vi "APC_9056_ArControl.vi"(1 "LoadIni?":bool, 3 "input cluster":T3={"AR-FT-001"=nan, "O2-FC-001"=-1.1539459916321034e-07, "SW-FT-004"=7.081032221378816e-08, "SW-FT-002"=-4.7206881475858774e-08, "WF-OA-002"=0.4443584404854535, "WF-PT-004"=nan, "WF-OA-001"=0.4434660166344514, "EC-TT-001"=2293.7171636993767, "WF-TT-004"=2293.7171636993767, "EC-FC-001"=0.0, "NG-FC-001"=-6.294250863447837e-08, "EO-TT-001"=2293.5316367979103, "SW-FC-008"=nan, "SW-FC-004"=0.0, "IMEPn6"=1.91605028485912e-05, "TORQUE"=0.44243251168443165, "CylPresWarnings"=5.764607523039514e+17, "CylPresErrors"=0.0, "NG-FT-001"=-1.3899803990113974e-07, "EngineSpeed_rpm"=0.0}) -> (0 "AR-PC-002-REF":dbl format="%.2f")   [LabVIEW 2020]
uses:
  controls/APC_PIDCluster.ctl
  controls/APC_ControlSettings.ctl
  controls/APC_PIDcontrolSettings.ctl
  controls/APC_cascadePIDsettings.ctl
  <vilib>/addons/control/pid/pid.llb/PID Advanced (DBL).vi
  <vilib>/Utility/xml.llb/Read From XML File(string).vi
  <vilib>/Utility/xml.llb/Write to XML File(string).vi
  <vilib>/addons/control/pid/NI_PID_pid.lvlib
panel:
  in  "PC_ControlSettings":T1={"Spark advance [CADBTDC]"=0.0, "Pref"=0.0, "O2ref"=0.0, "DI advance [CADBTDC]"=0.0, "DI duration [ms] "=0.0, "CO2ref"=0.0, "PFI duration [ms]"=0.0, "IMEP ref"=0.0, "Speed ref"=1800.0, "IGN enable"=TRUE, "DI enable"=TRUE, "CL PFI\n lambda"=FALSE, "CL PFI\nIMEP"=FALSE, "Activate\ncylinder"=[FALSE, FALSE, FALSE, FALSE, FALSE, FALSE], "Force idling"=FALSE, "Force motoring"=FALSE, "ETP resync"=FALSE, "Requested mode"=0, "Clear Sync Errors"=FALSE, "toggle TDC"=FALSE, "l ref"=0.0, "PID control references"={"NG"=FALSE, "Ar"=FALSE, "O2"=FALSE, "Intake vent"=FALSE, "Cross vent"=FALSE, "Exhaust vent"=FALSE, "NG control mode"=0, "NG-FC-001-REF"=0.0, "WF-OA-002-REF"=0.0, "IMEP-REF"=0.0, "Nm-REF"=0.0, "Ar control mode"=0, "AR-PC-002-REF"=0.0, "WF-PT-004-REF"=0.0, "O2 control mode"=0, "O2-FC-001-REF"=0.0, "WF-OA-001-REF"=0.0, "Tcoolant control  mode"=0, "EC-FC-001-REF"=0.0, "EC-TT-001-REF"=0.0, "Texh control mode"=0, "SW-FC-004-REF"=0.0, "SW-FT-002-REF"=0.0, "WF-TT-004-REF"=0.0, "Toil control mode"=0, "SW-FC-009-REF"=0.0, "SW-FT-004-REF"=0.0, "EO-TT-001-REF"=0.0, "AIC201_CO2_ConcTarget"=0.0, "O2_FF_NG"=FALSE, "Dyno control mode"=0, "Membrane control mode"=0, "AR-FT-001-REF"=0.0, "MTR modbus floats"=[0.0, 0.0, 0.0, 0.0, 0.0, 0.0, 0.0, 0.0, 0.0, 0.0, 0.0, 0.0, 0.0, 0.0, 0.0, 0.0, 0.0, 0.0, 0.0], "MTR modbus u16"=[0, 0, 0, 0, 0, 0, 0], "MTR HB"=FALSE, "PC_HB"=FALSE, "EMERGENCY STOP"=FALSE}, "CA50setpoint [CADATDC]"=0.0, "CA50 control"=TRUE, "Knock control"=FALSE, "CLEAR EMERGENCY STOP"=FALSE, "EMERGENCY STOP"=FALSE}
  out "PID control references.Ar":bool
  out "direct?":bool
  in  "AR-PC-002-REF (manual)":dbl
  out "Direct control":dbl=50.0 format="%.2f"
  in  "save":bool
  in  "load":bool
  out "Ar control mode":u8=2
  out "AR-FT-001":dbl=-1.0490418105746395e-08
  in  "LL FF control":dbl format="%.2f"
  in  "reinitialize LL? (F)":bool
  out "WF-PT-004":dbl=2293.8148612417403
  in  "SW-FT-001-REF (manual)":dbl
  in  "WF-PT-004-REF (manual)":dbl
  in  "Ar control mode (manual)":u8
  out "HL on?":bool
  out "HL setpoint":dbl=400.0 format="%.2f"
  in  "LL PID gains":T4 {"derivative time (Td, min)" format="%.3f"; "integral time (Ti, min)" format="%.3f"; "proportional gain (Kc)" format="%.3f"}
  in  "LL PID setpoint range":cluster{"setpoint high":dbl, "setpoint low":dbl} {"setpoint high" format="%.2f"; "setpoint low" format="%.2f"}
  in  "LL PID output range":cluster{"output high":dbl, "output low":dbl} {"output low" format="%.2f"; "output high" format="%.2f"}
  in  "Override PC PID references":bool
  in  "HL learn?":bool
  in  "HL FF control":dbl format="%.2f"
  in  "HL PID gains":T4 {"derivative time (Td, min)" format="%.3f"; "integral time (Ti, min)" format="%.3f"; "proportional gain (Kc)" format="%.3f"}
  in  "HL PID setpoint range":cluster{"setpoint high":dbl, "setpoint low":dbl} {"setpoint high" format="%.2f"; "setpoint low" format="%.2f"}
  in  "HL PID output range":cluster{"output high":dbl, "output low":dbl} {"output low" format="%.2f"; "output high" format="%.2f"}
  in  "Safe mode control":dbl format="%.2f"
  in  "LL learn?":bool
  in  "reinitialize HL? (F)":bool
  out "LL on?":bool=TRUE
  out "LL setpoint":dbl=40.0 format="%.2f"
  # "Ar control"
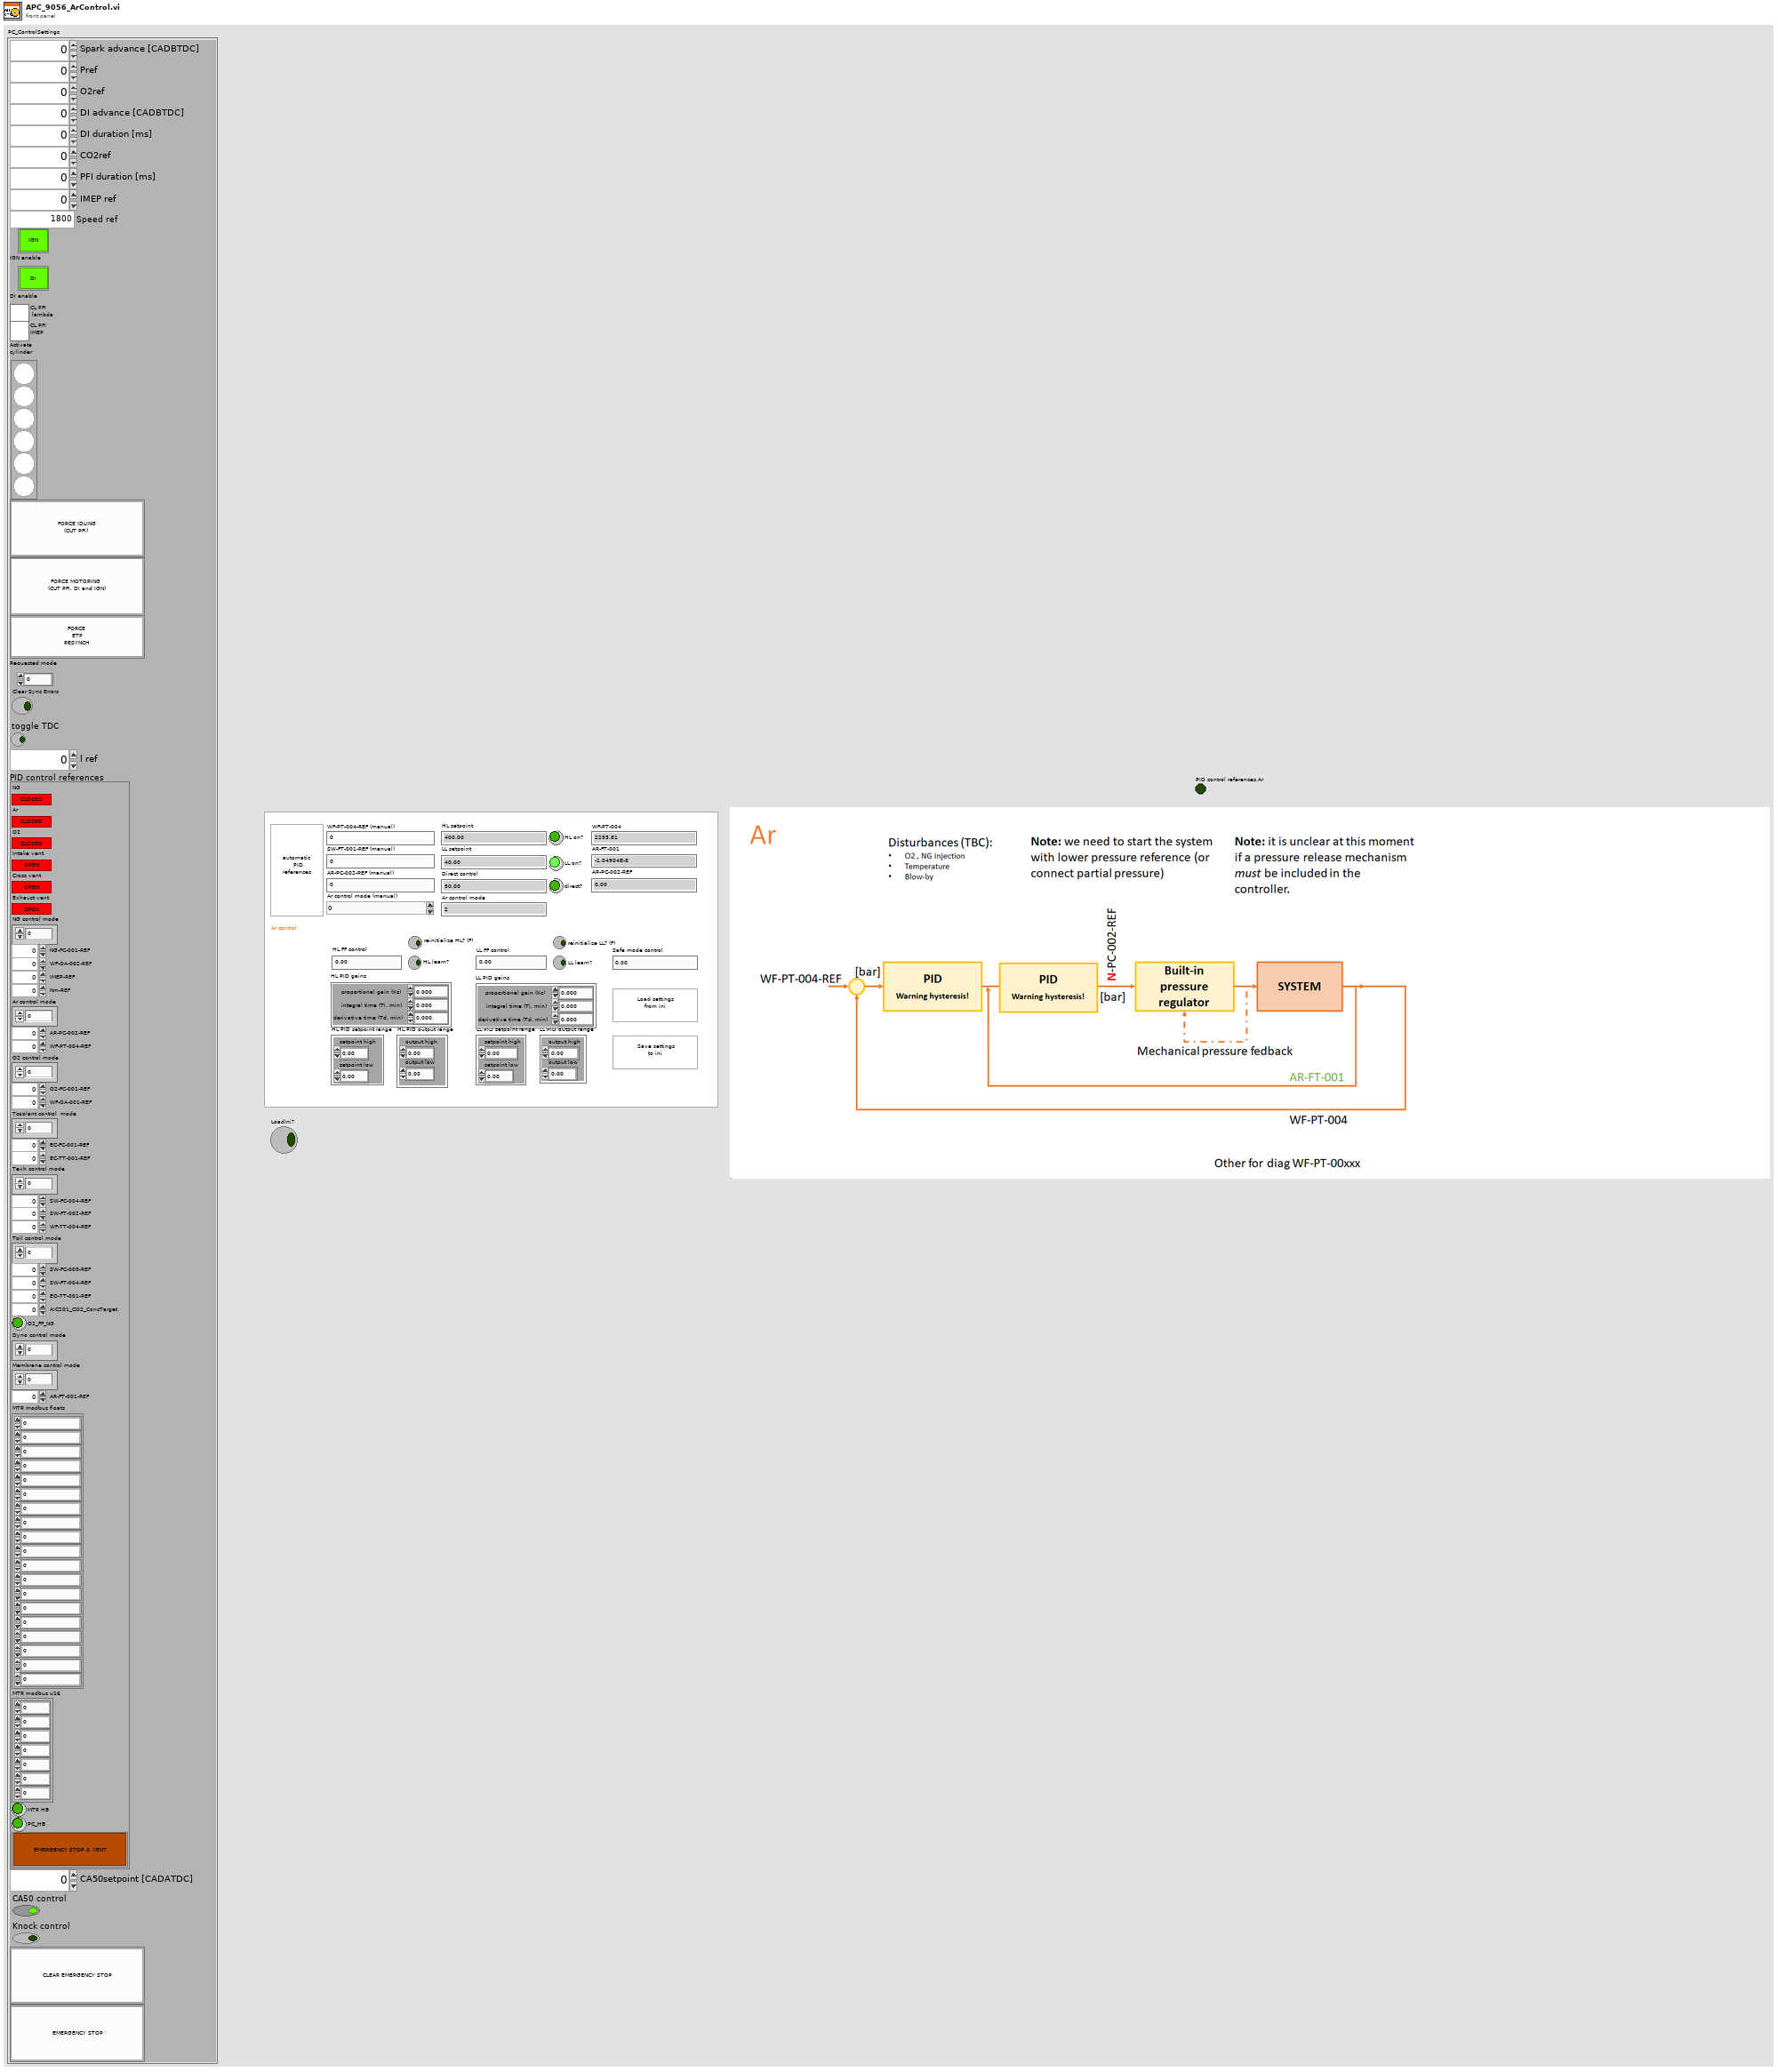
[diagram p1: front panel]
types:
  T1 = typedef "APC_ControlSettings.ctl" = cluster{"Spark advance [CADBTDC]":dbl, "Pref":dbl, "O2ref":dbl, "DI advance [CADBTDC]":dbl, "DI duration [ms] ":dbl, "CO2ref":dbl, "PFI duration [ms]":dbl, "IMEP ref":dbl, "Speed ref":dbl, "IGN enable":bool, "DI enable":bool, "CL PFI\n lambda":bool, "CL PFI\nIMEP":bool, "Activate\ncylinder":bool[], "Force idling":bool, "Force motoring":bool, "ETP resync":bool, "Requested mode":i8, "Clear Sync Errors":bool, "toggle TDC":bool, "l ref":dbl, "PID control references":T2, "CA50setpoint [CADATDC]":dbl, "CA50 control":bool, "Knock control":bool, "CLEAR EMERGENCY STOP":bool, "EMERGENCY STOP":bool}
  T2 = typedef "APC_PIDcontrolSettings.ctl" = cluster{"NG":bool, "Ar":bool, "O2":bool, "Intake vent":bool, "Cross vent":bool, "Exhaust vent":bool, "NG control mode":u8, "NG-FC-001-REF":dbl, "WF-OA-002-REF":dbl, "IMEP-REF":dbl, "Nm-REF":dbl, "Ar control mode":u8, "AR-PC-002-REF":dbl, "WF-PT-004-REF":dbl, "O2 control mode":u8, "O2-FC-001-REF":dbl, "WF-OA-001-REF":dbl, "Tcoolant control  mode":u8, "EC-FC-001-REF":dbl, "EC-TT-001-REF":dbl, "Texh control mode":u8, "SW-FC-004-REF":dbl, "SW-FT-002-REF":dbl, "WF-TT-004-REF":dbl, "Toil control mode":u8, "SW-FC-009-REF":dbl, "SW-FT-004-REF":dbl, "EO-TT-001-REF":dbl, "AIC201_CO2_ConcTarget":dbl, "O2_FF_NG":bool, "Dyno control mode":u8, "Membrane control mode":u8, "AR-FT-001-REF":dbl, "MTR modbus floats":sgl[], "MTR modbus u16":u16[], "MTR HB":bool, "PC_HB":bool, "EMERGENCY STOP":bool}
  T3 = typedef "APC_PIDCluster.ctl" = cluster{"AR-FT-001":dbl, "O2-FC-001":dbl, "SW-FT-004":dbl, "SW-FT-002":dbl, "WF-OA-002":dbl, "WF-PT-004":dbl, "WF-OA-001":dbl, "EC-TT-001":dbl, "WF-TT-004":dbl, "EC-FC-001":dbl, "NG-FC-001":dbl, "EO-TT-001":dbl, "SW-FC-008":dbl, "SW-FC-004":dbl, "IMEPn6":dbl, "TORQUE":dbl, "CylPresWarnings":dbl, "CylPresErrors":dbl, "NG-FT-001":dbl, "EngineSpeed_rpm":dbl}
  T4 = cluster{"proportional gain (Kc)":dbl, "integral time (Ti, min)":dbl, "derivative time (Td, min)":dbl}
  T5 = typedef "APC_cascadePIDsettings.ctl" = cluster{"HL FF control":dbl, "LL FF control":dbl, "HL PID gains":cluster{"proportional gain (Kc)":dbl, "integral time (Ti, min)":dbl, "derivative time (Td, min)":dbl}, "LL PID gains":cluster{"proportional gain (Kc)":dbl, "integral time (Ti, min)":dbl, "derivative time (Td, min)":dbl}, "HL PID setpoint range":cluster{"setpoint high":dbl, "setpoint low":dbl}, "HL PID output range":cluster{"output high":dbl, "output low":dbl}, "LL PID setpoint range":cluster{"setpoint high":dbl, "setpoint low":dbl}, "LL PID output range":cluster{"output high":dbl, "output low":dbl}, "Safe mode control":dbl}
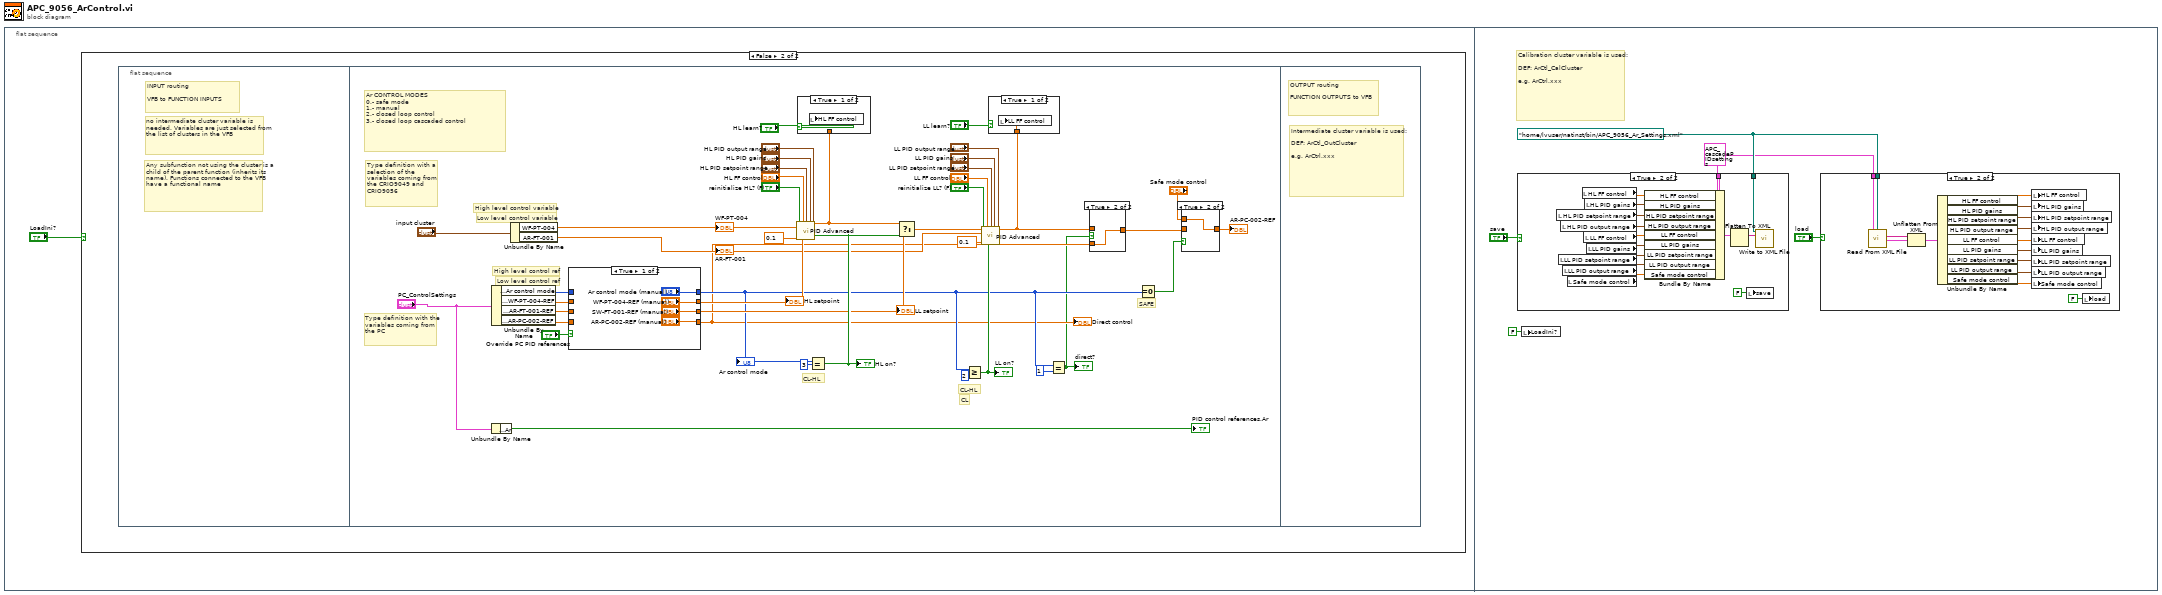
[diagram p0: block diagram]
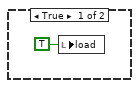
[diagram p2: hidden frame]
diagram:
  n1 = flat-sequence {
    frame #0 {
      n2 = case shown="False" "LoadIni?" {
        frame True {
          n3 = local write "load"(TRUE ("load")) -> ()
        }
        frame False {
          n4 = flat-sequence {
            frame #0 {
              # "Any subfunction not using the cluster is a child of the parent function (inherits its name). Functions connected to the VFB have a functional name"
              # "no intermediate cluster variable is needed. Variables are just selected from the list of clusters in the VFB"
              # "INPUT routing\n\nVFB to FUNCTION INPUTS"
            }
            frame #1 {
              # "Type definition with a selection of the variables coming from the CRIO9049 and CRIO9056"
              # "Type definition with the variables coming from the PC"
              # "CL-HL"
              # "Low level control ref"
              # "Low level control variable"
              # "High level control ref"
              # "High level control variable"
              # "SAFE"
              # "CL-HL"
              # "CL"
              # "Ar CONTROL MODES\n0.- safe mode\n1.- manual\n2.- closed loop control \n3.- closed loop cascaded control"
              n5 = Unbundle By Name("PC_ControlSettings") -> ("PID control references.Ar"=→"PID control references.Ar":bool)
              n6 = Unbundle By Name("PC_ControlSettings") -> ("PID control references.Ar control mode"=w21:u8, "PID control references.WF-PT-004-REF"=w20:dbl, "PID control references.AR-FT-001-REF"=w19:dbl, "PID control references.AR-PC-002-REF"=w7:dbl)
              n7 = Unbundle By Name("input cluster") -> ("WF-PT-004"=w18:dbl, "AR-FT-001"=w14:dbl)
              "WF-PT-004" <- w18
              "AR-FT-001" <- w14
              n8 = case shown="True" "Override PC PID references" {
                tunnel: w21 -> [_ w57]
                tunnel: w20 -> [_ w56]
                tunnel: w19 -> [_ w55]
                tunnel: ["Ar control mode (manual)" w57] -> w8
                tunnel: ["WF-PT-004-REF (manual)" w56] -> w17
                tunnel: ["SW-FT-001-REF (manual)" w55] -> w16
                tunnel: ["AR-PC-002-REF (manual)" w54] -> w6
                tunnel: w7 -> [_ w54]
                frame True {
                }
                frame False {
                }
              }
              "LL setpoint" <- w16
              "HL setpoint" <- w17
              "Ar control mode" <- w8
              "Direct control" <- w6
              n9 = Equal?(x=w8, y=u8 3) -> (x = y?=w27:bool)
              "HL on?" <- w27
              n10 = call-poly <vilib>:"PID Advanced.vi"("setpoint"=w17, "output range"="HL PID output range", "auto? (T)"=w27, "manual control"="HL FF control", "process variable"=w18, "setpoint range"="HL PID setpoint range", "PID gains"="HL PID gains", "dt (s)"=0.1, "reinitialize? (F)"="reinitialize HL? (F)") -> ("output"=w32:dbl)  [unwired: 5 in, 1 out]
              n11 = case shown="True" "HL learn?" {
                tunnel: w32 -> [w49 _]
                frame True {
                  n12 = local write "HL FF control"(w49) -> ()
                }
                frame False {
                }
              }
              n13 = Select(t=w32, s=w27, f=w16) -> (s? t:f=w38:dbl)
              n14 = Greater Or Equal?(x=w8, y=u8 2) -> (x >= y?=w41:bool)
              "LL on?" <- w41
              n15 = call-poly <vilib>:"PID Advanced.vi"("setpoint"=w38, "output range"="LL PID output range", "auto? (T)"=w41, "manual control"="LL FF control", "process variable"=w14, "setpoint range"="LL PID setpoint range", "PID gains"="LL PID gains", "dt (s)"=0.1, "reinitialize? (F)"="reinitialize LL? (F)") -> ("output"=w10:dbl)  [unwired: 5 in, 1 out]
              n16 = case shown="True" "LL learn?" {
                tunnel: w10 -> [w46 _]
                frame True {
                  n17 = local write "LL FF control"(w46) -> ()
                }
                frame False {
                }
              }
              n18 = Equal?(x=w8, y=u8 1) -> (x = y?=w5:bool)
              "direct?" <- w5
              n19 = case shown="True" w5 {
                tunnel: [w44 w45] -> w9
                tunnel: w10 -> [w44 _]
                tunnel: w6 -> [_ w45]
                frame False {
                }
                frame True {
                }
              }
              n20 = Equal To 0?(x=w8) -> (x = 0?=w43:bool)
              n21 = case shown="True" w43 {
                tunnel: [w47 w48] -> w26
                tunnel: "Safe mode control" -> [_ w48]
                tunnel: w9 -> [w47 _]
                frame False {
                }
                frame True {
                }
              }
              "AR-PC-002-REF" <- w26
            }
            frame #2 {
              # "Intermediate cluster variable is used:\n\nDEF: ArCtl_OutCluster\n\ne.g. ArCtrl.xxx"
              # "OUTPUT routing\n\nFUNCTION OUTPUTS to VFB"
            }
          }
        }
      }
    }
    frame #1 {
      w60 = path "/home/lvuser/natinst/bin/APC_9056_Ar_Settings.xml" ("XML File Path")
      w59 = T5 {"HL FF control"=0.0, "LL FF control"=0.0, "HL PID gains"={"proportional gain (Kc)"=1.0, "integral time (Ti, min)"=0.01, "derivative time (Td, min)"=0.0}, "LL PID gains"={"proportional gain (Kc)"=1.0, "integral time (Ti, min)"=0.01, "derivative time (Td, min)"=0.0}, "HL PID setpoint range"={"setpoint high"=100.0, "setpoint low"=0.0}, "HL PID output range"={"output high"=0.0, "output low"=0.0}, "LL PID setpoint range"={"setpoint high"=100.0, "setpoint low"=0.0}, "LL PID output range"={"output high"=10.0, "output low"=-10.0}, "Safe mode control"=0.0} ("Cluster")
      # "Calibration cluster variable is used:\n\nDEF: ArCtl_CalCluster\n\ne.g. ArCtrl.xxx"
      n22 = case shown="True" "save" {
        tunnel: w60 -> [_ w79]
        tunnel: w59 -> [_ w78]
        frame False {
        }
        frame True {
          n23 = local read "HL PID setpoint range"() -> (w88:cluster{"setpoint high":dbl, "setpoint low":dbl})
          n24 = local read "LL PID setpoint range"() -> (w84:cluster{"setpoint high":dbl, "setpoint low":dbl})
          n25 = local read "HL PID output range"() -> (w87:cluster{"output high":dbl, "output low":dbl})
          n26 = local read "LL PID output range"() -> (w83:cluster{"output high":dbl, "output low":dbl})
          n27 = local read "Safe mode control"() -> (w82:dbl)
          n28 = local read "HL FF control"() -> (w90:dbl)
          n29 = local read "LL FF control"() -> (w86:dbl)
          n30 = local read "HL PID gains"() -> (w89:T4)
          n31 = local read "LL PID gains"() -> (w85:T4)
          n32 = Bundle By Name(cluster=w78, "HL FF control"=w90, "HL PID gains"=w89, "HL PID setpoint range"=w88, "HL PID output range"=w87, "LL FF control"=w86, "LL PID gains"=w85, "LL PID setpoint range"=w84, "LL PID output range"=w83, "Safe mode control"=w82) -> (w81:T5)
          n33 = Flatten To XML(6:w81) -> (2:w80:string)
          n34 = local write "save"(FALSE ("load")) -> ()
          n35 = call-poly <vilib>:"Write to XML File.vi"("XML Input"=w80, "XML File Path"=w79) -> ()  [unwired: 7 in, 3 out]
        }
      }
      n36 = local write "LoadIni?"(FALSE ("LoadIni?")) -> ()
      n37 = case shown="True" "load" {
        tunnel: w60 -> [_ w75]
        tunnel: w59 -> [_ w74]
        frame False {
        }
        frame True {
          n38 = call-poly <vilib>:"Read From XML File.vi"("XML File Path"=w75) -> ("XML Elements"=w76:string)  [unwired: 8 in, 2 out]
          n39 = Unflatten From XML(xml string=w76, type=w74) -> (value=w73:T5)  [unwired: 1 in, 1 out]
          n40 = Unbundle By Name(w73) -> ("HL FF control"=w72:dbl, "HL PID gains"=w71:T4, "HL PID setpoint range"=w70:cluster{"setpoint high":dbl, "setpoint low":dbl}, "HL PID output range"=w69:cluster{"output high":dbl, "output low":dbl}, "LL FF control"=w68:dbl, "LL PID gains"=w67:T4, "LL PID setpoint range"=w66:cluster{"setpoint high":dbl, "setpoint low":dbl}, "LL PID output range"=w65:cluster{"output high":dbl, "output low":dbl}, "Safe mode control"=w64:dbl)
          n41 = local write "HL FF control"(w72) -> ()
          n42 = local write "HL PID gains"(w71) -> ()
          n43 = local write "HL PID setpoint range"(w70) -> ()
          n44 = local write "HL PID output range"(w69) -> ()
          n45 = local write "LL FF control"(w68) -> ()
          n46 = local write "LL PID gains"(w67) -> ()
          n47 = local write "LL PID setpoint range"(w66) -> ()
          n48 = local write "LL PID output range"(w65) -> ()
          n49 = local write "Safe mode control"(w64) -> ()
          n50 = local write "load"(FALSE ("save")) -> ()
        }
      }
    }
  }
